vi "Doppler Moving STFT PtByPt.vi"() -> ()   [LabVIEW 2022 SP3]
doc: "Performs real-time Joint Time Frequency Analysis (JTFA) using Point By Point STFT. The signal is simulated by a sine wave plus Gaussian noise."
uses:
  <vilib>/measure/mamon.llb/Waveform Peak Detection for N Chan.vi
  <vilib>/ptbypt/NI_PtbyPt.lvlib
  <vilib>/Analysis/NI_AALPro.lvlib
  <vilib>/measure/NI_MAPro.lvlib
panel:
  out "# data pts":i32
  out "Waveform Graph 4":dynamicdata(graph)
  out "Waveform Graph 3":dbl[](graph)
  out "Waveform Graph 2":dbl[](graph)
  out "locations time 1":dbl[](array[numeric])
  out "locations time 0":dbl[](array[numeric])
  out "Locations":cluster{"Locations":dbl[]}[](array[cluster]) {"Locations" format="%.2p"}
  out "Amplitudes":cluster{"Amplitudes":dbl[]}[](array[cluster]) {"Amplitudes" format="%.2p"}
  out "# peaks found":i32[](array[numeric])
  out "Waveform Graph":dbl[][](graph)
  out "Array 3":dbl[][](array[numeric])
  out "DT":dbl
  out "dt":dbl
  out "Number of cols (freq)":dbl
  out "Number of rows (time)":dbl
  out "Array 2":i32[](array[numeric])
  out "Boolean 2":bool
  in  "time increment":i32=200
  out "Boolean":bool
  out "Doppler signal":dynamicdata(graph) caption="Signals"
  out "Moving STFT":dbl[][](graph)
  in  "sample length":i32=200
  in  "window length":i32=100 format="%0.0f"
  in  "stop":bool
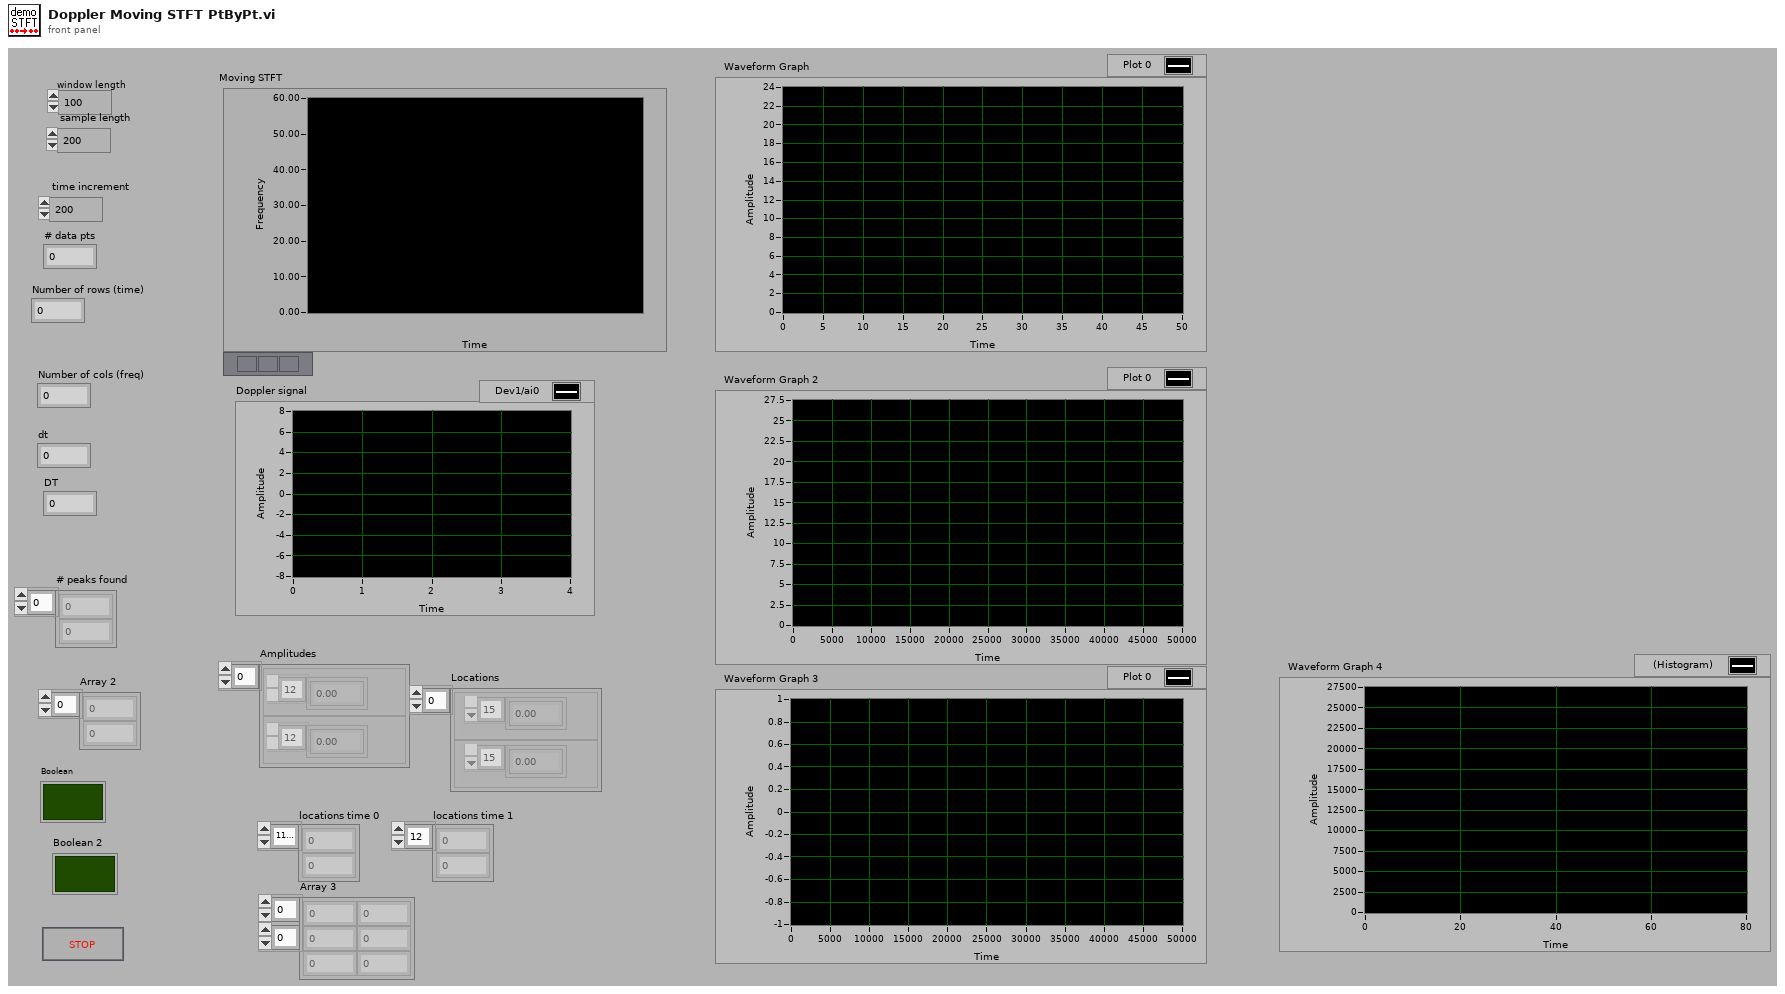
[diagram p1: front panel]
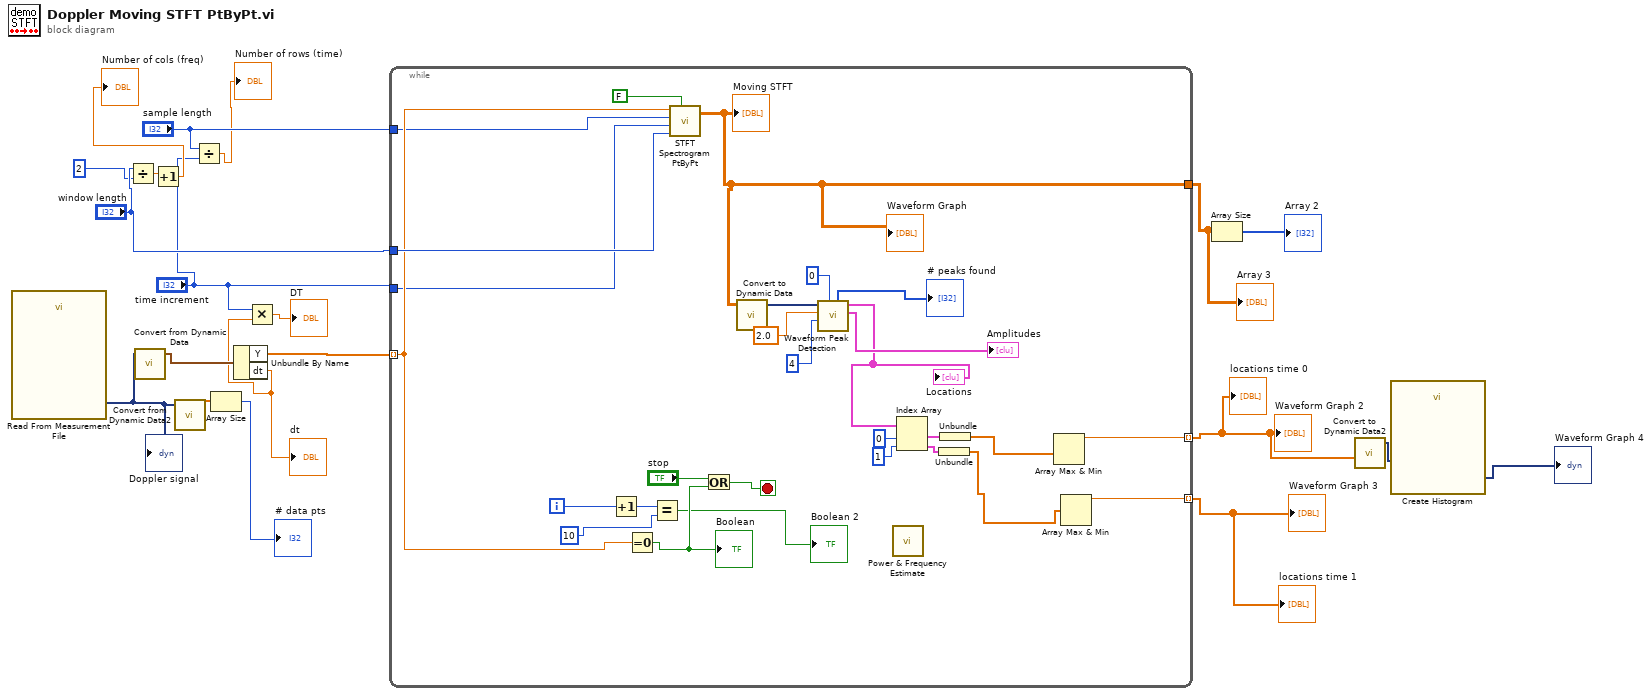
[diagram p0: block diagram]
diagram:
  n1 = call "Read From Measurement File"() -> ("Signals"=w17:dynamicdata)  [unwired: 4 in, 7 out]
  "Doppler signal" <- w17
  n2 = Divide(x="window length", y=u32 2 ("milliseconds to wait")) -> (x/y=w13:dbl)
  n3 = call "Convert from Dynamic Data"("Dynamic Data Type"=w17) -> ("Waveform"=w18:waveform(dbl))  [unwired: 1 in, 2 out]
  n4 = Increment(x=w13) -> (x+1=→"Number of cols (freq)":dbl)
  n5 = call "Convert from Dynamic Data2"("Dynamic Data Type"=w17) -> ("Array"=w16:dbl[])  [unwired: 3 out]
  n6 = Divide(x="sample length", y="time increment") -> (x/y=→"Number of rows (time)":dbl)
  n7 = Array Size(array=w16) -> (size(s)=→"# data pts":i32)
  n8 = Unbundle By Name(w18) -> ("Y"=w20:dbl[], "dt"=w7:dbl)
  "dt" <- w7
  n9 = Multiply(x="time increment", y=w7) -> (x*y=→"DT":dbl)
  n10 = while {
    tunnel: "window length" -> [w48]
    tunnel: w20 -> [w47] mode=indexing
    tunnel: "time increment" -> [w44]
    tunnel: "sample length" -> [w39]
    tunnel: [w36] -> w6
    tunnel: [w22] -> w4 mode=indexing
    tunnel: [w21] -> w5 mode=indexing
    i -> [w38]
    stop <- w45 stop-if-true
    n11 = Increment(x=w38) -> (x+1=w43:i32)
    n12 = Equal To 0?(x=w47) -> (x = 0?=w41:bool)
    "Boolean" <- w41
    n13 = Equal?(x=w43, y=u32 10 ("milliseconds to wait")) -> (x = y?=→"Boolean 2":bool)
    n14 = call <vilib>:"STFT Spectrogram PtByPt.vi"("initialize"=FALSE, "window length"=w48, "time increment"=w44, "sample length"=w39, "x"=w47) -> ("STFT Spectrogram {X}"=w36:dbl[][])  [unwired: 1 in, 1 out]
    "Moving STFT" <- w36
    "Waveform Graph" <- w36
    n15 = Or(x="stop", y=w41) -> (x .or. y?=w45:bool)
    n16 = call "Convert to Dynamic Data"("2D Array"=w36) -> ("Dynamic Data Type"=w35:dynamicdata)  [unwired: 3 out]
    n17 = call-poly <vilib>:"Waveform Peak Detection.vi"("peaks/valleys"=u32 0 ("milliseconds to wait"), "width"=u32 4 ("milliseconds to wait"), "threshold"=2.0 ("Y Scale.Range:Minimum"), "Signals In"=w35) -> ("Amplitudes"=→"Amplitudes":cluster{"Amplitudes":dbl[]}[], "Locations"=w29:cluster{"Locations":dbl[]}[], "# found"=→"# peaks found":i32[])  [unwired: 3 in, 2 out]
    "Locations" <- w29
    n18 = call <vilib>:"Power & Frequency Estimate.vi"() -> ()  [unwired: 5 in, 3 out]
    n19 = Index Array(array=w29, index #1=u32 0 ("milliseconds to wait"), index #2=u32 1 ("milliseconds to wait")) -> (element #1=w27:cluster{"Locations":dbl[]}, element #2=w25:cluster{"Locations":dbl[]})
    n20 = Unbundle(w25) -> ("Locations"=w23:dbl[])
    n21 = Unbundle(w27) -> ("Locations"=w24:dbl[])
    n22 = Array Max & Min(array=w24) -> (max value=w22:dbl)  [unwired: 3 out]
    n23 = Array Max & Min(array=w23) -> (max value=w21:dbl)  [unwired: 3 out]
  }
  "Array 3" <- w6
  "Waveform Graph 2" <- w4
  "Waveform Graph 3" <- w5
  "locations time 0" <- w4
  "locations time 1" <- w5
  n24 = Array Size(array=w6) -> (size(s)=→"Array 2":i32[])
  n25 = call "Convert to Dynamic Data2"("Array"=w4) -> ("Dynamic Data Type"=w3:dynamicdata)  [unwired: 3 out]
  n26 = call "Create Histogram"("Signal"=w3) -> ("Histogram"=→"Waveform Graph 4":dynamicdata)  [unwired: 3 in, 7 out]
